vi "build_XML_string.vi"(5 "xml declaration":string="<?xml version=\"1.0\" encoding='UTF-8'?>", 6 "pretty print?":bool, 7 "ID tag":string="ID", 8 "error in (no error)":errorcluster, 11 "Element in":refnum<class "XMLElement.lvclass">) -> (0 "error out":errorcluster, 2 "string":string, 3 "Element out":refnum<class "XMLElement.lvclass">)   [LabVIEW 2010, in "XMLElement.lvclass"]
uses:
  XMLElement.lvclass
  XMLElement.lvclass/XMLElement.ctl
  Program Files/National Instruments/LabVIEW 2010/resource/objmgr/DOMUserDefRef.rc
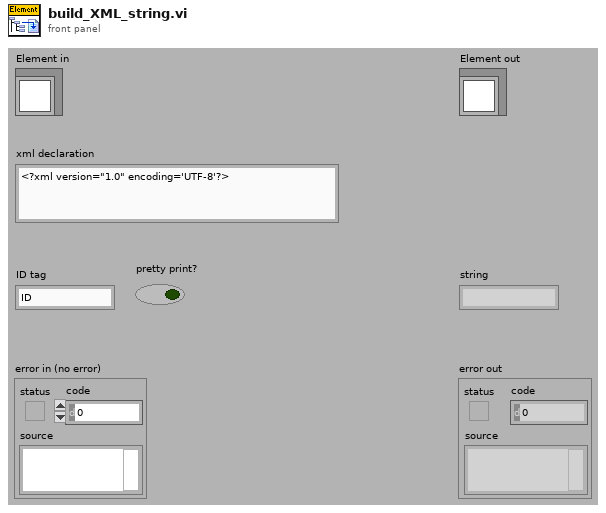
[diagram p1: front panel]
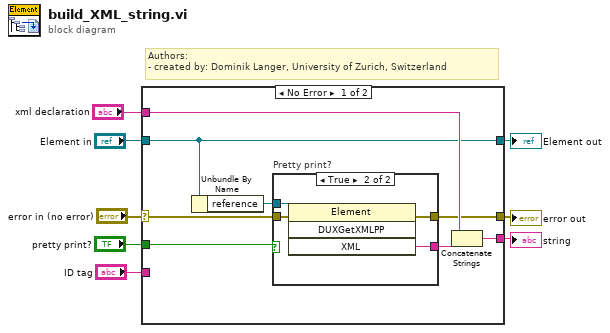
[diagram p0: block diagram]
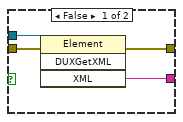
[diagram p2: hidden frame]
diagram:
  # "Authors: \n- created by: Dominik Langer, University of Zurich, Switzerland"
  n1 = case shown="No Error" "error in (no error)" {
    selector: "error in (no error)" -> [w12 w26]
    tunnel: [w11 w26] -> w7
    tunnel: [w14 w25] -> w5
    tunnel: "Element in" -> [w14 w25]
    tunnel: "ID tag" -> [_ _]
    tunnel: "xml declaration" -> [w15 _]
    tunnel: [w16 _] -> w2
    tunnel: "pretty print?" -> [w9 _]
    frame No Error {
      n2 = Unbundle By Name(w14) -> ("reference"=w13:refnum<k20>)
      n3 = case "Pretty print?" shown="True" w9 {
        tunnel: w13 -> [w20 w24]
        tunnel: w12 -> [w19 w23]
        tunnel: [w18 w22] -> w11
        tunnel: [w17 w21] -> w10
        frame False {
          n4 = invoke class="Element" method="DUXGetXML"(reference=w20, error in=w19) -> (error out=w18:errorcluster, "XML"=w17:string)  [unwired: 2 in, 2 out]
        }
        frame True {
          n5 = invoke class="Element" method="DUXGetXMLPP"(reference=w24, error in=w23) -> (error out=w22:errorcluster, "XML"=w21:string)  [unwired: 2 in, 2 out]
        }
      }
      n6 = Concatenate Strings(w15, w10) -> (w16:string)
    }
    frame Error {
    }
  }
  "error out" <- w7
  "Element out" <- w5
  "string" <- w2
